vi "Get Control Label.vi"(0 "Control In":refnum<vi>, 1 "error in (no error)":errorcluster) -> (2 "Control Out":refnum<vi>, 3 "Text":string, 4 "error out":errorcluster)   [LabVIEW 2012, in "Scripting Tools.lvlib"]
doc: "Returns the label of the control passed by reference."
uses:
  Scripting Tools.lvlib
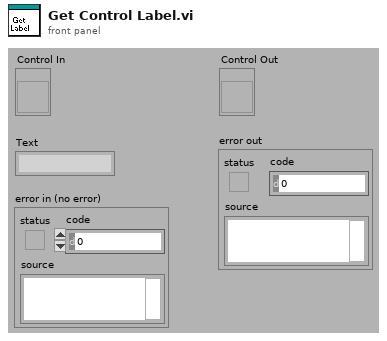
[diagram p1: front panel]
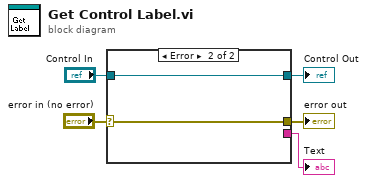
[diagram p0: block diagram]
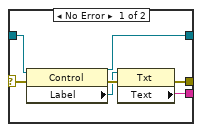
[diagram p2: hidden frame]
diagram:
  n1 = case shown="Error" "error in (no error)" {
    selector: "error in (no error)" -> [w6 w14]
    tunnel: [w10 _] -> w5
    tunnel: "Control In" -> [w9 w13]
    tunnel: [w8 w13] -> w3
    tunnel: [w7 w14] -> w2
    frame No Error {
      n2 = property class="Control"(reference=w9, error in=w6) -> (reference out=w8:refnum<vi>, error out=w12:errorcluster, "Label"=w11:refnum<vi>)
      n3 = property class="Txt"(reference=w11, error in=w12) -> (error out=w7:errorcluster, "Text"=w10:string)  [unwired: 1 out]
    }
    frame Error {
    }
  }
  "Text" <- w5
  "Control Out" <- w3
  "error out" <- w2
